vi "TCPsendCommand.vi"(0 "DashboardServer in":refnum<class "Dashboard Server.lvclass">, 1 "command":string, 2 "data":string, 5 "error in (no error)":errorcluster, 8 "add delay (T)":bool=TRUE) -> (14 "DashboardServer out":refnum<class "Dashboard Server.lvclass">, 15 "returnStatus":string, 16 "data":string, 19 "error out":errorcluster)   [LabVIEW 2019, in "Dashboard Server.lvclass"]
uses:
  Dashboard Server.lvclass
  Dashboard Server.lvclass/Dashboard Server.ctl
  <vilib>/Utility/error.llb/whitespace.ctl
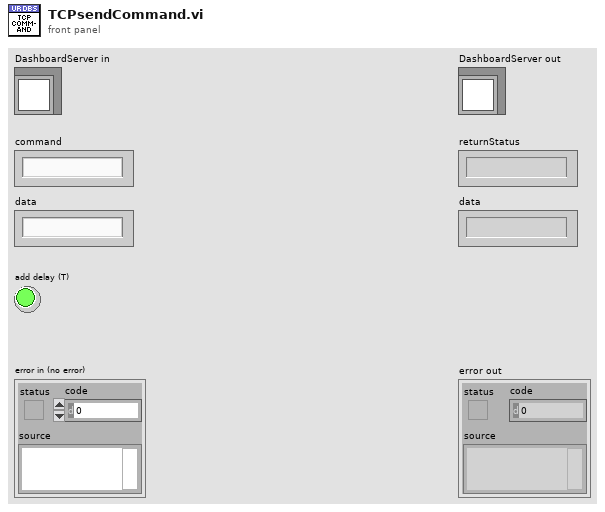
[diagram p1: front panel]
types:
  T1 = enum16{"Standard", "Buffered", "CRLF", "Immediate"}
  T2 = typedef "whitespace.ctl" = u16
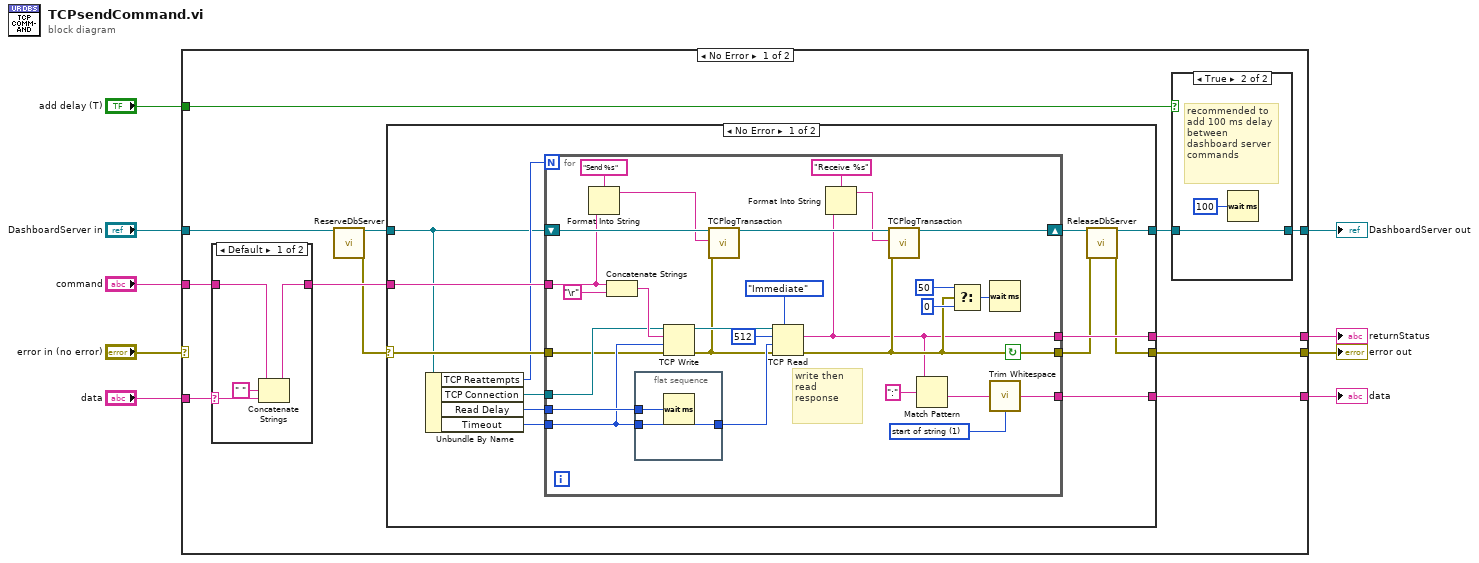
[diagram p0: block diagram]
diagram:
  n1 = case shown="No Error" "error in (no error)" {
    selector: "error in (no error)" -> [_ w76]
    tunnel: [w13 w76] -> w9
    tunnel: [w11 w75] -> w8
    tunnel: "DashboardServer in" -> [w20 w75]
    tunnel: "command" -> [w16 _]
    tunnel: [w18 _] -> w6
    tunnel: [w21 _] -> w7
    tunnel: "data" -> [w17 _]
    tunnel: "add delay (T)" -> [w10 _]
    frame No Error {
      n2 = case shown="Default" w17 {
        selector: w17 -> [w72 _]
        tunnel: w16 -> [w73 w74]
        tunnel: [w71 w74] -> w15
        frame Default {
          n3 = Concatenate Strings(w73, " " ("string"), w72) -> (w71:string)
        }
        frame "" {
        }
      }
      n4 = call "ReserveDbServer.vi"("DashboardServer in"=w20) -> ("DashboardServer out"=w19:refnum<class "Dashboard Server.lvclass">, "error out"=w14:errorcluster)  [unwired: 17 in]
      n5 = case shown="No Error" w14 {
        selector: w14 -> [w30 w68]
        tunnel: [w34 _] -> w21
        tunnel: w19 -> [w25 w69]
        tunnel: [w33 w69] -> w12
        tunnel: [w32 _] -> w18
        tunnel: w15 -> [w31 _]
        tunnel: [w28 w68] -> w13
        frame No Error {
          n6 = Unbundle By Name(w25) -> ("TCP Reattempts"=w27:i32, "TCP Connection"=w37:refnum<k5>, "Read Delay"=w36:u32, "Timeout"=w35:i32)
          n7 = for {
            N: w27 -> [_]
            tunnel: w37 -> [w60]
            tunnel: w36 -> [w58]
            tunnel: w35 -> [w57]
            tunnel: [w39] -> w34
            tunnel: [w53] -> w32
            tunnel: w31 -> [w43]
            tunnel: w30 -> [w52]
            tunnel: [w46] -> w29
            shift-right: [w45] -> w26
            shift-left: w25 -> [w44]
            stop <- w46 continue-if-true
            w54 = T2 1 items=["both", "start of string", "end of string"] ("location (both)")
            # "write then read response"
            n8 = Format Into String(format string="Send %s", w43) -> (resulting string=w42:string)  [unwired: 2 in, 1 out]
            n9 = Concatenate Strings(w43, "\r") -> (w62:string)
            n10 = flat-sequence {
              tunnel: w58 -> [w67]
              tunnel: w57 -> [w66]
              tunnel: [w66] -> w56
              frame #0 {
                n11 = Wait (ms)(milliseconds to wait=w67) -> ()  [unwired: 1 out]
              }
            }
            n12 = TCP Write(connection ID=w60, data in=w62, error in (no error)=w52, 9:w57) -> (connection ID out=w59:refnum<k5>, error out=w48:errorcluster)  [unwired: 1 out]
            n13 = call "TCPlogTransaction.vi"("Dashboard Server in"=w44, "Transaction"=w42, "error in (no error)"=w48) -> ("Dashboard Server out"=w47:refnum<class "Dashboard Server.lvclass">)  [unwired: 16 in]
            n14 = TCP Read(connection ID=w59, bytes to read=512, error in (no error)=w48, 7:T1."Immediate" ("mode (standard)"), 9:w56) -> (data out=w39:string, error out=w46:errorcluster)  [unwired: 1 out]
            n15 = Format Into String(format string="Receive %s", w39) -> (resulting string=w38:string)  [unwired: 2 in, 1 out]
            n16 = call "TCPlogTransaction.vi"("Dashboard Server in"=w47, "Transaction"=w38, "error in (no error)"=w46) -> ("Dashboard Server out"=w45:refnum<class "Dashboard Server.lvclass">)  [unwired: 16 in]
            n17 = Match Pattern(string=w39, regular expression=":") -> (after substring=w55:string)  [unwired: 1 in, 3 out]
            n18 = Select(t=u32 50, s=w46, f=u32 0 ("milliseconds to wait")) -> (s? t:f=w50:u32)
            n19 = Wait (ms)(milliseconds to wait=w50) -> ()  [unwired: 1 out]
            n20 = call <vilib>:"Trim Whitespace.vi"("string"=w55, "location (both)"=w54) -> ("trimmed string"=w53:string)
          }
          n21 = call "ReleaseDbServer.vi"("DashboardServer in"=w26, "error in (no error)"=w29) -> ("DashboardServer out"=w33:refnum<class "Dashboard Server.lvclass">, "error out"=w28:errorcluster)  [unwired: 16 in]
        }
        frame Error {
          # "unable to reserve reference"
        }
      }
      n22 = case shown="True" w10 {
        tunnel: w12 -> [w22 w24]
        tunnel: [w22 w24] -> w11
        frame False {
        }
        frame True {
          # "recommended to add 100 ms delay between dashboard server commands"
          n23 = Wait (ms)(milliseconds to wait=u32 100) -> ()  [unwired: 1 out]
        }
      }
    }
    frame Error {
    }
  }
  "error out" <- w9
  "DashboardServer out" <- w8
  "returnStatus" <- w7
  "data" <- w6
